vi "M TV WT RC.vi"(11 "NXT/EV3":T1) -> (3 "EV3 out":T1)   [LabVIEW 2016]
uses:
  <vilib>/NXT/Subs/LVHSConnector.ctl
  <vilib>/NXT/LegoClasses/BrickReference/BrickReference.lvclass
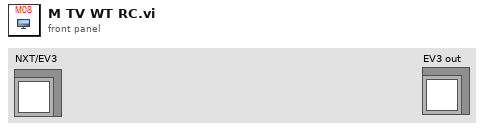
[diagram p1: front panel]
types:
  T1 = typedef "LVHSConnector.ctl" = refnum<class "BrickReference.lvclass">
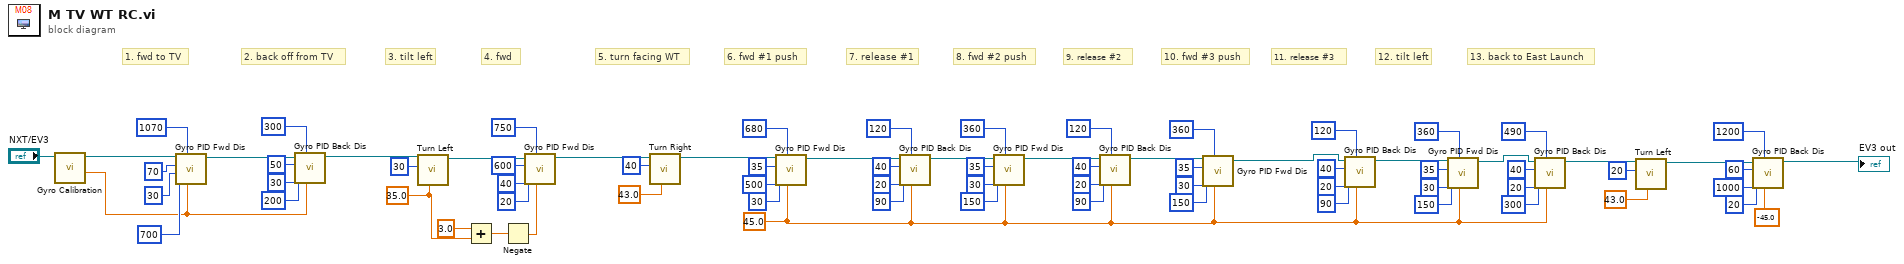
[diagram p0: block diagram]
diagram:
  w1 = sgl 45.0 ("Target angle")
  w58 = sgl 35.0 ("Turning angle")
  # "13. back to East Launch"
  # "12. tilt left"
  # "11. release #3"
  # "10. fwd #3 push"
  # "9. release #2"
  # "8. fwd #2 push"
  # "7. release #1"
  # "6. fwd #1 push"
  # "5. turn facing WT"
  # "4. fwd"
  # "3. tilt left"
  # "2. back off from TV"
  # "1. fwd to TV"
  n1 = call "Gyro Calibration.vi"("NXT/EV3"="NXT/EV3") -> ("Degrees"=w66:sgl, "NXT/EV3"=w77:T1)  [unwired: 6 in, 1 out]
  n2 = call "Gyro PID Fwd Dis.vi"("Target angle"=w66, "Threshold to stop"=1070, "Threshold to slow"=700, "Min. speed"=30, "Max. speed"=70, "EV3 in"=w77) -> ("EV3 out"=w71:T1)  [unwired: 5 in]
  n3 = call "Gyro PID Back Dis.vi"("Target angle"=w66, "Threshold to stop"=300, "Threshold to slow"=200, "Min. speed"=30, "Max. speed"=50, "EV3 in"=w71) -> ("EV3 out"=w65:T1)  [unwired: 5 in]
  n4 = call "Turn Left.vi"("Turning angle"=w58, "Motor B (right)"=i8 30, "EV3 in"=w65) -> ("EV3 out"=w63:T1)  [unwired: 8 in]
  n5 = Add(x=sgl 3.0, y=w58) -> (x+y=w56:sgl)
  n6 = Negate(x=w56) -> (-x=w55:sgl)
  n7 = call "Gyro PID Fwd Dis.vi"("Target angle"=w55, "Threshold to stop"=750, "Threshold to slow"=20, "Min. speed"=40, "Max. speed"=600, "EV3 in"=w63) -> ("EV3 out"=w54:T1)  [unwired: 5 in]
  n8 = call "Turn Right.vi"("Turning angle"=sgl 43.0, "Motor B (right)"=i8 40, "EV3 in"=w54) -> ("EV3 out"=w51:T1)  [unwired: 8 in]
  n9 = call "Gyro PID Fwd Dis.vi"("Target angle"=w1, "Threshold to stop"=680, "Threshold to slow"=30, "Min. speed"=500, "Max. speed"=35, "EV3 in"=w51) -> ("EV3 out"=w46:T1)  [unwired: 5 in]
  n10 = call "Gyro PID Back Dis.vi"("Target angle"=w1, "Threshold to stop"=120, "Threshold to slow"=90, "Min. speed"=20, "Max. speed"=40, "EV3 in"=w46) -> ("EV3 out"=w41:T1)  [unwired: 5 in]
  n11 = call "Gyro PID Fwd Dis.vi"("Target angle"=w1, "Threshold to stop"=360, "Threshold to slow"=150, "Min. speed"=30, "Max. speed"=35, "EV3 in"=w41) -> ("EV3 out"=w36:T1)  [unwired: 5 in]
  n12 = call "Gyro PID Back Dis.vi"("Target angle"=w1, "Threshold to stop"=120, "Threshold to slow"=90, "Min. speed"=20, "Max. speed"=40, "EV3 in"=w36) -> ("EV3 out"=w30:T1)  [unwired: 5 in]
  n13 = call "Gyro PID Fwd Dis.vi"("Target angle"=w1, "Threshold to stop"=360, "Threshold to slow"=150, "Min. speed"=30, "Max. speed"=35, "EV3 in"=w30) -> ("EV3 out"=w2:T1)  [unwired: 5 in]
  n14 = call "Gyro PID Back Dis.vi"("Target angle"=w1, "Threshold to stop"=120, "Threshold to slow"=90, "Min. speed"=20, "Max. speed"=40, "EV3 in"=w2) -> ("EV3 out"=w7:T1)  [unwired: 5 in]
  n15 = call "Gyro PID Fwd Dis.vi"("Target angle"=w1, "Threshold to stop"=360, "Threshold to slow"=150, "Min. speed"=30, "Max. speed"=35, "EV3 in"=w7) -> ("EV3 out"=w3:T1)  [unwired: 5 in]
  n16 = call "Gyro PID Back Dis.vi"("Target angle"=w1, "Threshold to stop"=490, "Threshold to slow"=300, "Min. speed"=20, "Max. speed"=40, "EV3 in"=w3) -> ("EV3 out"=w22:T1)  [unwired: 5 in]
  n17 = call "Turn Left.vi"("Turning angle"=sgl 43.0, "Motor B (right)"=i8 20, "EV3 in"=w22) -> ("EV3 out"=w19:T1)  [unwired: 8 in]
  n18 = call "Gyro PID Back Dis.vi"("Target angle"=sgl -45.0, "Threshold to stop"=1200, "Threshold to slow"=20, "Min. speed"=1000, "Max. speed"=60, "EV3 in"=w19) -> ("EV3 out"=→"EV3 out":T1)  [unwired: 5 in]
